vi "MecaWheelPos_Get.vi"(11 "MECA_WHEEL_POSITIONS":T1 {"RearRight" format="%19.3f"; "RearLeft" format="%19.3f"; "FrontRight" format="%19.3f"; "FrontLeft" format="%19.3f"}) -> (0 "RearRightPosition":dbl format="%19.3f", 1 "RearLeftPosition":dbl format="%19.3f", 2 "FrontRightPosition":dbl format="%19.3f", 3 "FrontLeftPosition":dbl format="%19.3f")   [LabVIEW 2019, in "Trajectory_Library.lvlib"]
doc: "Extract individual positions (distances) from a MecanumDriveWheelPosition data structure.\n\nParameters:\n - Meca_wheel_Position- Data structure\n\nReturns:\n - Left Front Position - Distance measured by left front wheel (meters)\n - Right Front Position - Distance measured by right front wheel (meters)\n - Left Rear Position - Distance measured by left rear wheel (meters)\n - Right Rear Position - Distance measured by right rear wheel (meters)"
uses:
  Trajectory_Library.lvlib
  TypeDef/MECA_WHEEL_POSITIONS.ctl
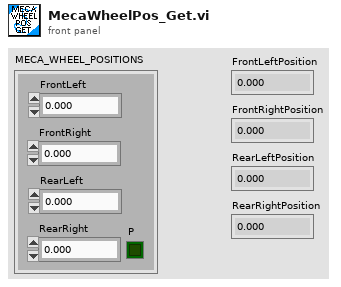
[diagram p1: front panel]
types:
  T1 = typedef "Trajectory_Library.lvlib/MECA_WHEEL_POSITIONS.ctl" = cluster{"FrontLeft":dbl, "FrontRight":dbl, "RearLeft":dbl, "RearRight":dbl, "P":bool}
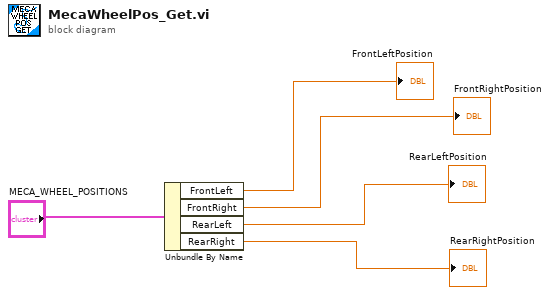
[diagram p0: block diagram]
diagram:
  n1 = Unbundle By Name("MECA_WHEEL_POSITIONS") -> ("FrontLeft"=→"FrontLeftPosition":dbl, "FrontRight"=→"FrontRightPosition":dbl, "RearLeft"=→"RearLeftPosition":dbl, "RearRight"=→"RearRightPosition":dbl)
